vi "ParcialSemaforo.vi"() -> ()   [LabVIEW 2023]
panel:
  out "Boolean 4":bool
  out "Boolean 3":bool
  out "Boolean 2":bool=TRUE
  in  "Boolean":bool
  # "Daniel Garzon\n\nLaura Herrera\n\nSebastian Rodriguez"
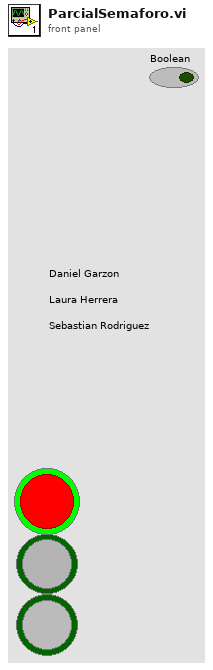
[diagram p1: front panel]
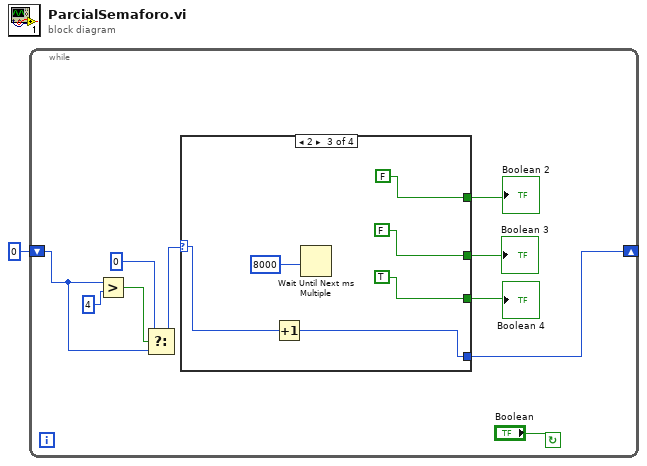
[diagram p0: block diagram]
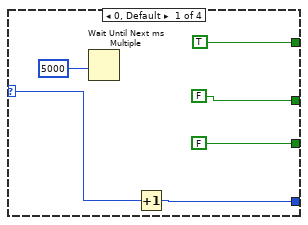
[diagram p2: hidden frame]
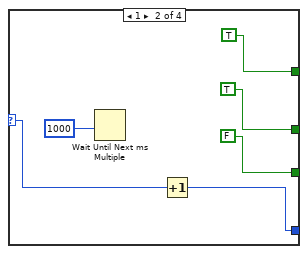
[diagram p3: hidden frame]
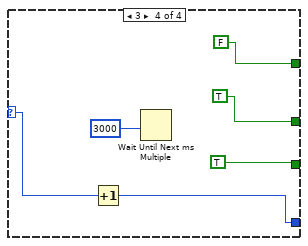
[diagram p4: hidden frame]
diagram:
  n1 = while {
    shift-right: [w7] -> _
    shift-left: 0 -> [w4]
    stop <- "Boolean" continue-if-true
    n2 = Greater?(x=w4, y=4) -> (0:w5:bool)
    n3 = Select(t=0, s=w5, f=w4) -> (s? t:f=w2:i32)
    n4 = case shown="2" w2 {
      selector: w2 -> [w13 w19 w25 w31]
      tunnel: [FALSE TRUE FALSE TRUE] -> w10
      tunnel: [FALSE FALSE TRUE TRUE] -> w9
      tunnel: [TRUE TRUE FALSE FALSE] -> w8
      tunnel: [w12 w18 w24 w30] -> w7
      frame 0, Default {
        n5 = Wait Until Next ms Multiple(millisecond multiple=5000) -> ()  [unwired: 1 out]
        n6 = Increment(x=w13) -> (x+1=w12:i32)
      }
      frame 1 {
        n7 = Wait Until Next ms Multiple(millisecond multiple=1000) -> ()  [unwired: 1 out]
        n8 = Increment(x=w19) -> (x+1=w18:i32)
      }
      frame 2 {
        n9 = Increment(x=w25) -> (x+1=w24:i32)
        n10 = Wait Until Next ms Multiple(millisecond multiple=8000) -> ()  [unwired: 1 out]
      }
      frame 3 {
        n11 = Increment(x=w31) -> (x+1=w30:i32)
        n12 = Wait Until Next ms Multiple(millisecond multiple=3000) -> ()  [unwired: 1 out]
      }
    }
    "Boolean 2" <- w8
    "Boolean 3" <- w10
    "Boolean 4" <- w9
  }
